vi "3D_Plot_Cursor_position.vi"(0 "3D Spectrum Plot":dbl[][](array[numeric]), 5 "3D Spectrum Cursor Pos X":dbl, 7 "3D Spectrum Cursor Pos Y":dbl, 9 "Wavelength":dbl[](array[numeric]), 11 "Delay Positions":dbl[](array[numeric])) -> (2 "Delay 3D CursorPosX":dbl, 3 "Delay 3D CursorPosY":dbl, 4 "Delay 3D":T1, 8 "Spectrum 3D":T2, 13 "Spectrum 3D CursorPosX":dbl, 14 "Spectrum 3D CursorPosY":dbl, 15 "Energy [eV]":dbl)   [LabVIEW 2009]
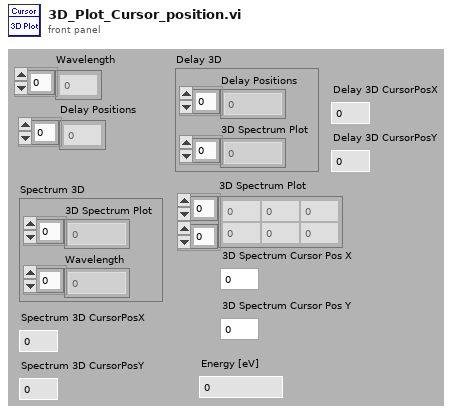
[diagram p1: front panel]
types:
  T1 = cluster{"Delay Positions":dbl[], "3D Spectrum Plot":dbl[]}
  T2 = cluster{"3D Spectrum Plot":dbl[], "Wavelength":dbl[]}
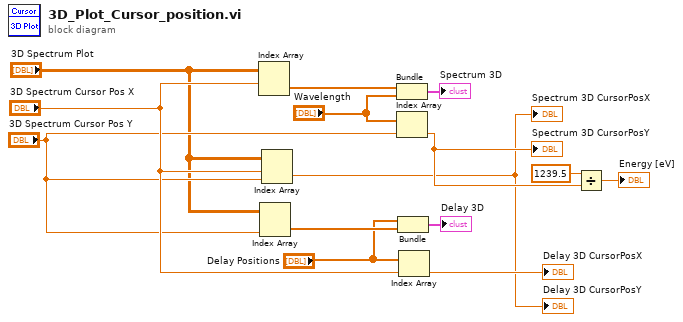
[diagram p0: block diagram]
diagram:
  n1 = Index Array(array="3D Spectrum Plot", index (row)="3D Spectrum Cursor Pos X") -> (element=w14:dbl[])  [unwired: 1 in]
  n2 = Index Array(array="3D Spectrum Plot", index (col)="3D Spectrum Cursor Pos Y") -> (element=w13:dbl[])  [unwired: 1 in]
  n3 = Index Array(array="3D Spectrum Plot", index (row)="3D Spectrum Cursor Pos X", index (col)="3D Spectrum Cursor Pos Y") -> (element=→"Spectrum 3D CursorPosX" →"Delay 3D CursorPosY":dbl)
  n4 = Bundle("3D Spectrum Plot"=w14, "Wavelength"="Wavelength") -> (→"Spectrum 3D":T2)  [unwired: 1 in]
  n5 = Index Array(array="Wavelength", index="3D Spectrum Cursor Pos Y") -> (element=w4:dbl)
  "Spectrum 3D CursorPosY" <- w4
  n6 = Bundle("Delay Positions"="Delay Positions", "3D Spectrum Plot"=w13) -> (→"Delay 3D":T1)  [unwired: 1 in]
  n7 = Index Array(array="Delay Positions", index="3D Spectrum Cursor Pos X") -> (element=→"Delay 3D CursorPosX":dbl)
  n8 = Divide(x=1239.5 ("y"), y=w4) -> (x/y=→"Energy [eV]":dbl)
